vi "Import LabVIEW.ini Tokens.vi"   [LabVIEW 2014]
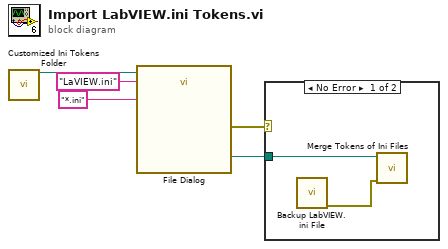
[diagram p0: block diagram]
diagram:
  n1 = call "Customized Ini Tokens Folder.vi"() -> ("appended path"=w3:path)  [unwired: 19 in]
  n2 = call "File Dialog"("start path"=w3, "default name"="LaVIEW.ini", "pattern (all files)"="*.ini") -> ("selected path"=w4:path, "error out"=w5:errorcluster)  [unwired: 9 in, 2 out]
  n3 = case shown="No Error" w5 {
    tunnel: w4 -> [w7 _]
    frame No Error {
      n4 = call "Backup LabVIEW.ini File.vi"() -> ("error out"=w6:errorcluster)  [unwired: 10 in, 1 out]
      n5 = call "Merge Tokens of Ini Files.vi"("error in (no error)"=w6, "Path"=w7) -> ()  [unwired: 9 in, 1 out]
    }
    frame Error {
    }
  }
